vi "PCO_GetAcquireControl.vi"(8 "error in (no error)":errorcluster {"code" format="%x"}, 11 "ph":u64) -> (0 "error out":errorcluster {"code" format="%x"}, 2 "ErrorMessage":i32 format="%x", 3 "ph out":u64)   [LabVIEW 2019, in "SDK.lvlib" / "RecordingControl.lvlib"]
doc: "<b>Description:</b>\nThis function sets the acquire mode of the camera.\nAcquire mode can be either [auto], [external] or [external modulate].\n\n<b>Supported camera type:</b>\nAll cameras\n\n<b>Descriptor dependency:</b>\ndwGeneralCapsDESC1: NO_ACQUIREMODE"
uses:
  RecordingControl.lvlib
panel:
  out "dwAcquCtrlFlags":u32(ring) items=["ACQUIRE_CONTROL_OFF", "ACQUIRE_CONTROL_FORCE_LOW", "ACQUIRE_CONTROL_FORCE_HIGH"]
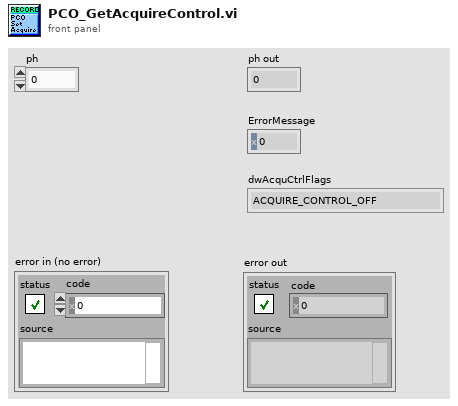
[diagram p1: front panel]
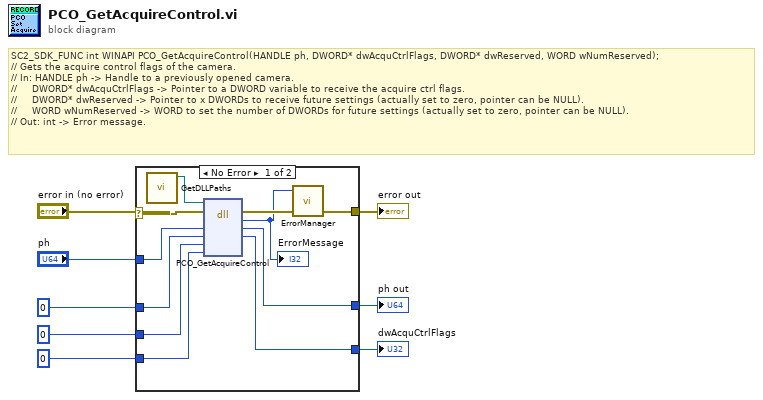
[diagram p0: block diagram]
diagram:
  # "SC2_SDK_FUNC int WINAPI PCO_GetAcquireControl(HANDLE ph, DWORD* dwAcquCtrlFlags, DWORD* dwReserved, WORD wNumReserved);\n// Gets the acquire control flags of the camera.\n// In: HANDLE ph -> Handle to a previously opened camera.\n//     DWORD* dwAcquCtrlFlags -> Pointer to a DWORD variable to receive the acquire ctrl flags.\n//     DWORD* dwReserved -> Pointer to x DWORDs to receive future settings (actually set to zero, pointer can be NULL).\n//     WORD wNumReserved -> WORD to set the number of DWORDs for future settings (actually set to zero, pointer can be NULL).\n// Out: int -> Error message."
  n1 = case shown="No Error" "error in (no error)" {
    selector: "error in (no error)" -> [w16 w22]
    tunnel: "ph" -> [w19 w21]
    tunnel: [w18 w21] -> w7
    tunnel: u32 0 ("dwAcquCtrlFlags") -> [w17 w20]
    tunnel: [w14 w22] -> w6
    tunnel: u32 0 -> [w11 _]
    tunnel: u16 0 -> [w10 _]
    tunnel: [w9 w20] -> w1
    frame No Error {
      n2 = call "GetDLLPaths.vi"() -> ("SC2_Cam_Path"=w12:path)  [unwired: 9 in, 2 out]
      n3 = dll-call lib="?" fn="PCO_GetAcquireControl"(path in=w12, error in=w16, "ph"=w19, "dwAcquCtrlFlags"=w17, "dwReserved"=w11, "wNumReserved"=w10) -> (error out=w15:errorcluster, "return type"=w13:i32, "ph"=w18:u64, "dwAcquCtrlFlags"=w9:u32)  [unwired: 3 in, 1 out]
      "ErrorMessage" <- w13
      n4 = call "ErrorManager.vi"("error in (no error)"=w15, "error code"=w13) -> ("error out"=w14:errorcluster)  [unwired: 3 in]
    }
    frame Error {
    }
  }
  "ph out" <- w7
  "dwAcquCtrlFlags" <- w1
  "error out" <- w6
